vi "InitCSMs.vi"(8 "error in (no error)":errorcluster, 11 "testcase-CSMSyncMessage in":refnum<class "testcase-CSMSyncMessage.lvclass">) -> (0 "error out":errorcluster, 3 "testcase-CSMSyncMessage out":refnum<class "testcase-CSMSyncMessage.lvclass">)   [LabVIEW 2017, in "testcase-CSMSyncMessage.lvclass"]
uses:
  testcase-CSMSyncMessage.lvclass
  testcase-CSMSyncMessage.lvclass/testcase-CSMSyncMessage.ctl
  CSM/Chain1.vi
  <vilib>/AppBuilder/AB_API_Simple/Build (path).vi
  CSM/CSM-Testcase.lvlib
  src/user.lib/_NEVSTOP/Communicable State Machine(CSM)/Communicable State Machine.lvlib
  <vilib>/AppBuilder/AB_API_Simple/NI_App_Builder_API.lvlib
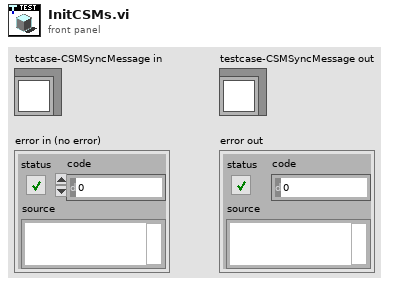
[diagram p1: front panel]
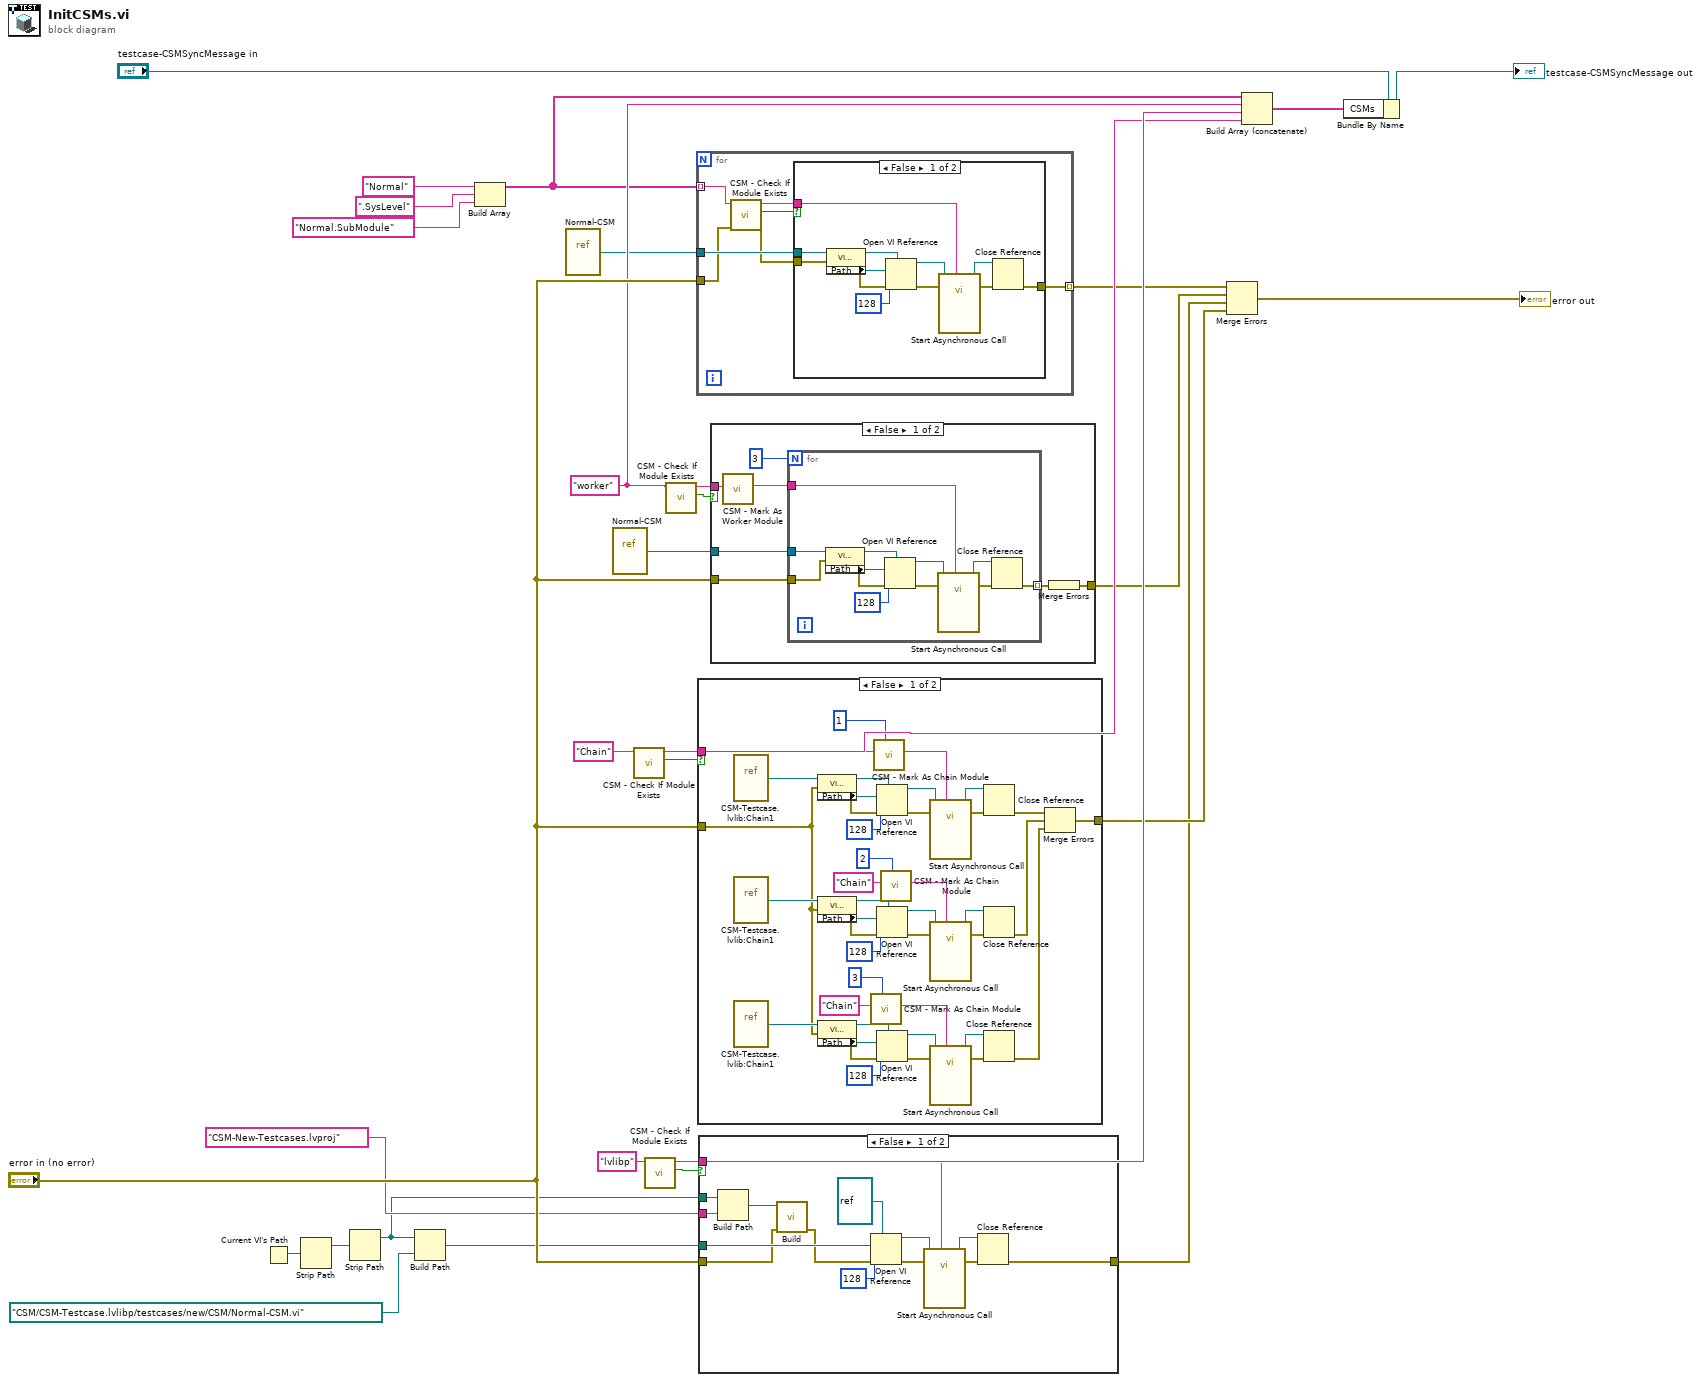
[diagram p0: block diagram]
diagram:
  w23 = "worker" ("Name (\"\" to Use UUID)")
  n1 = Current VI's Path() -> (path=w14:path)
  n2 = Strip Path(path=w14) -> (stripped path=w17:path)  [unwired: 1 out]
  n3 = Strip Path(path=w17) -> (stripped path=w18:path)  [unwired: 1 out]
  n4 = Build Path(base path=w18, name or relative path=path "CSM/CSM-Testcase.lvlibp/testcases/new/CSM/Normal-CSM.vi" ("vi path")) -> (appended path=w16:path)
  n5 = Build Array("Normal" ("Name (\"\" to Use UUID)"), ".SysLevel" ("Name (\"\" to Use UUID)"), "Normal.SubModule" ("Name (\"\" to Use UUID)")) -> (w7:string[])
  n6 = vi-ref "Normal-CSM.vi"() -> (w3:refnum<vi>)
  n7 = vi-ref "Normal-CSM.vi"() -> (w10:refnum<vi>)
  n8 = call "CSM - Check If Module Exists.vi"("CSM Name"="Chain" ("Name (\"\" to Use UUID)")) -> ("Exist?"=w27:bool, "CSM Name (Dup)"=w26:string)  [unwired: 8 in, 1 out]
  n9 = call "CSM - Check If Module Exists.vi"("CSM Name"="lvlibp" ("Name (\"\" to Use UUID)")) -> ("Exist?"=w30:bool, "CSM Name (Dup)"=w28:string)  [unwired: 8 in, 1 out]
  n10 = call "CSM - Check If Module Exists.vi"("CSM Name"=w23) -> ("Exist?"=w25:bool, "CSM Name (Dup)"=w24:string)  [unwired: 8 in, 1 out]
  n11 = for {
    tunnel: w3 -> [w37]
    tunnel: w7 -> [w33] mode=indexing
    tunnel: [w36] -> w8 mode=indexing
    tunnel: "error in (no error)" -> [w35]
    n12 = call "CSM - Check If Module Exists.vi"("Error In"=w35, "CSM Name"=w33) -> ("error out"=w34:errorcluster, "Exist?"=w31:bool, "CSM Name (Dup)"=w32:string)  [unwired: 7 in]
    n13 = case shown="False" w31 {
      tunnel: w37 -> [w41 _]
      tunnel: [w40 w50] -> w36
      tunnel: w34 -> [w39 w50]
      tunnel: w32 -> [w38 _]
      frame False {
        n14 = property class="VI (strict)"(reference=w41, error in=w39) -> (reference out=w47:refnum<vi>, error out=w45:errorcluster, "Path"=w44:path)
        n15 = Open VI Reference(type specifier VI Refnum (for type only)=w47, vi path=w44, options=128, error in (no error)=w45) -> (vi reference=w43:refnum<vi>, error out=w48:errorcluster)  [unwired: 2 in]
        n16 = call-by-ref "Start Asynchronous Call"(reference=w43, error in=w48, "Name (\"\" to Use UUID)"=w38) -> (reference out=w42:refnum<vi>, error out=w46:errorcluster)  [unwired: 11 in]
        n17 = Close Reference(reference=w42, error in (no error)=w46) -> (error out=w40:errorcluster)
      }
      frame True {
      }
    }
  }
  n18 = case shown="False" w27 {
    tunnel: [w53 w92] -> w22
    tunnel: "error in (no error)" -> [w52 w92]
    tunnel: w26 -> [w51 _]
    frame False {
      n19 = vi-ref "CSM-Testcase.lvlib:Chain1.vi"() -> (w91:refnum<vi>)
      n20 = vi-ref "CSM-Testcase.lvlib:Chain1.vi"() -> (w74:refnum<vi>)
      n21 = vi-ref "CSM-Testcase.lvlib:Chain1.vi"() -> (w71:refnum<vi>)
      n22 = property class="VI (strict)"(reference=w91, error in=w52) -> (reference out=w88:refnum<vi>, error out=w86:errorcluster, "Path"=w85:path)
      n23 = property class="VI (strict)"(reference=w74, error in=w52) -> (reference out=w77:refnum<vi>, error out=w79:errorcluster, "Path"=w80:path)
      n24 = property class="VI (strict)"(reference=w71, error in=w52) -> (reference out=w68:refnum<vi>, error out=w66:errorcluster, "Path"=w65:path)
      n25 = call "CSM - Mark As Chain Module.vi"("Order"=3, "CSM Name"="Chain" ("Name (\"\" to Use UUID)")) -> ("CSM Name (Marked As Chain)"=w59:string)  [unwired: 8 in]
      n26 = call "CSM - Mark As Chain Module.vi"("Order"=1, "CSM Name"=w51) -> ("CSM Name (Marked As Chain)"=w57:string)  [unwired: 8 in]
      n27 = Open VI Reference(type specifier VI Refnum (for type only)=w88, vi path=w85, options=128, error in (no error)=w86) -> (vi reference=w84:refnum<vi>, error out=w89:errorcluster)  [unwired: 2 in]
      n28 = Open VI Reference(type specifier VI Refnum (for type only)=w77, vi path=w80, options=128, error in (no error)=w79) -> (vi reference=w81:refnum<vi>, error out=w76:errorcluster)  [unwired: 2 in]
      n29 = Open VI Reference(type specifier VI Refnum (for type only)=w68, vi path=w65, options=128, error in (no error)=w66) -> (vi reference=w64:refnum<vi>, error out=w69:errorcluster)  [unwired: 2 in]
      n30 = call "CSM - Mark As Chain Module.vi"("Order"=2, "CSM Name"="Chain" ("Name (\"\" to Use UUID)")) -> ("CSM Name (Marked As Chain)"=w58:string)  [unwired: 8 in]
      n31 = call-by-ref "Start Asynchronous Call"(reference=w84, error in=w89, "Name (\"\" to Use UUID)"=w57) -> (reference out=w83:refnum<vi>, error out=w87:errorcluster)  [unwired: 11 in]
      n32 = call-by-ref "Start Asynchronous Call"(reference=w81, error in=w76, "Name (\"\" to Use UUID)"=w58) -> (reference out=w82:refnum<vi>, error out=w78:errorcluster)  [unwired: 11 in]
      n33 = call-by-ref "Start Asynchronous Call"(reference=w64, error in=w69, "Name (\"\" to Use UUID)"=w59) -> (reference out=w63:refnum<vi>, error out=w67:errorcluster)  [unwired: 11 in]
      n34 = Close Reference(reference=w83, error in (no error)=w87) -> (error out=w62:errorcluster)
      n35 = Close Reference(reference=w82, error in (no error)=w78) -> (error out=w61:errorcluster)
      n36 = Close Reference(reference=w63, error in (no error)=w67) -> (error out=w60:errorcluster)
      n37 = Merge Errors(w62, w61, w60) -> (w53:errorcluster)
    }
    frame True {
    }
  }
  n38 = case shown="False" w30 {
    tunnel: [w106 w107] -> w13
    tunnel: w16 -> [w99 _]
    tunnel: w18 -> [w98 _]
    tunnel: "CSM-New-Testcases.lvproj" ("name or relative path") -> [w96 _]
    tunnel: w28 -> [w95 _]
    tunnel: "error in (no error)" -> [w94 w107]
    frame False {
      n39 = Build Path(base path=w98, name or relative path=w96) -> (appended path=w97:path)
      n40 = call-poly <vilib>:"Build.vi"("error in (no error)"=w94, "Path to project"=w97) -> ("error out"=w93:errorcluster)  [unwired: 8 in, 1 out]
      n41 = Open VI Reference(type specifier VI Refnum (for type only)=refnum<vi> refnum ("reference out"), vi path=w99, options=128, error in (no error)=w93) -> (vi reference=w102:refnum<vi>, error out=w104:errorcluster)  [unwired: 2 in]
      n42 = call-by-ref "Start Asynchronous Call"(reference=w102, error in=w104, "Name (\"\" to Use UUID)"=w95) -> (reference out=w101:refnum<vi>, error out=w103:errorcluster)  [unwired: 11 in]
      n43 = Close Reference(reference=w101, error in (no error)=w103) -> (error out=w106:errorcluster)
    }
    frame True {
    }
  }
  n44 = case shown="False" w25 {
    tunnel: w10 -> [w114 _]
    tunnel: [w108 w127] -> w11
    tunnel: "error in (no error)" -> [w110 w127]
    tunnel: w24 -> [w109 _]
    frame False {
      n45 = call "CSM - Mark As Worker Module.vi"("CSM Name"=w109) -> ("CSM Name (Marked As Worker)"=w111:string)  [unwired: 9 in]
      n46 = for {
        N: 3 -> [_]
        tunnel: w114 -> [w118]
        tunnel: w111 -> [w117]
        tunnel: [w116] -> w112 mode=indexing
        tunnel: w110 -> [w115]
        n47 = property class="VI (strict)"(reference=w118, error in=w115) -> (reference out=w124:refnum<vi>, error out=w122:errorcluster, "Path"=w121:path)
        n48 = Open VI Reference(type specifier VI Refnum (for type only)=w124, vi path=w121, options=128, error in (no error)=w122) -> (vi reference=w120:refnum<vi>, error out=w125:errorcluster)  [unwired: 2 in]
        n49 = call-by-ref "Start Asynchronous Call"(reference=w120, error in=w125, "Name (\"\" to Use UUID)"=w117) -> (reference out=w119:refnum<vi>, error out=w123:errorcluster)  [unwired: 11 in]
        n50 = Close Reference(reference=w119, error in (no error)=w123) -> (error out=w116:errorcluster)
      }
      n51 = Merge Errors(w112) -> (w108:errorcluster)
    }
    frame True {
    }
  }
  n52 = Merge Errors(w8, w11, w13, w22) -> (→"error out":errorcluster)
  n53 = Build Array (concatenate)(w7, w23, w28, w26) -> (w12:string[])
  n54 = Bundle By Name(cluster="testcase-CSMSyncMessage in", "CSMs"=w12) -> (→"testcase-CSMSyncMessage out":refnum<class "testcase-CSMSyncMessage.lvclass">)
